vi "CRYGraph Get.vi"(11 "pGraph VI In":refnum<vi>) -> (3 "Graph Cluster":T1)   [LabVIEW 2013]
uses:
  Control/CRYGraph Property.ctl
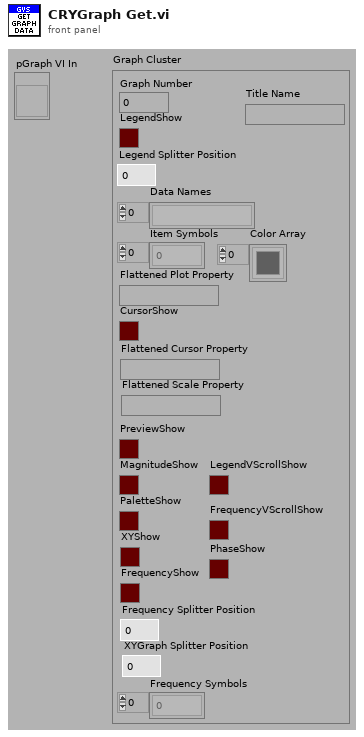
[diagram p1: front panel]
types:
  T1 = typedef "CRYGraph Property.ctl" = cluster{"LegendShow":bool, "Legend Splitter Position":dbl, "Data Names":string[], "Item Symbols":i32[], "Color Array":u32[], "Flattened Plot Property":string, "CursorShow":bool, "Flattened Cursor Property":string, "Graph Number":i32, "Flattened Scale Property":string, "PreviewShow":bool, "MagnitudeShow":bool, "PaletteShow":bool, "XYShow":bool, "FrequencyShow":bool, "Frequency Splitter Position":dbl, "XYGraph Splitter Position":dbl, "Frequency Symbols":i32[], "LegendVScrollShow":bool, "FrequencyVScrollShow":bool, "PhaseShow":bool, "Title Name":string}
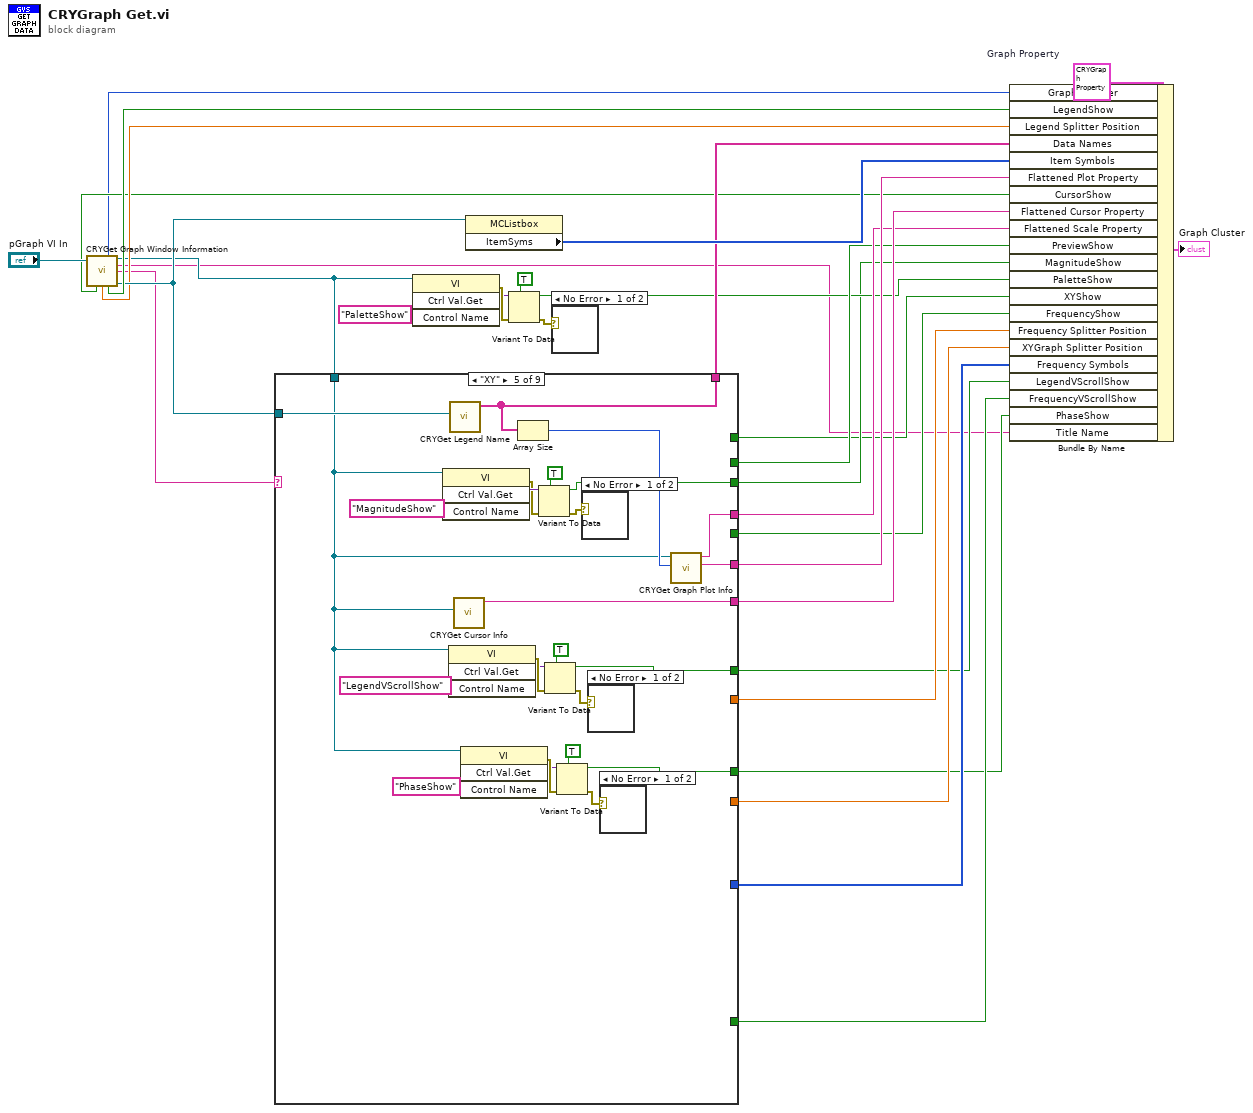
[diagram p0: block diagram]
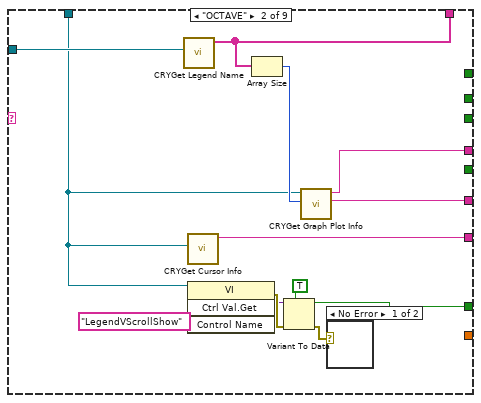
[diagram p4: hidden frame]
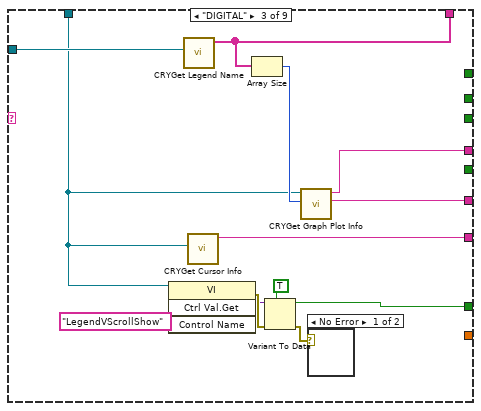
[diagram p6: hidden frame]
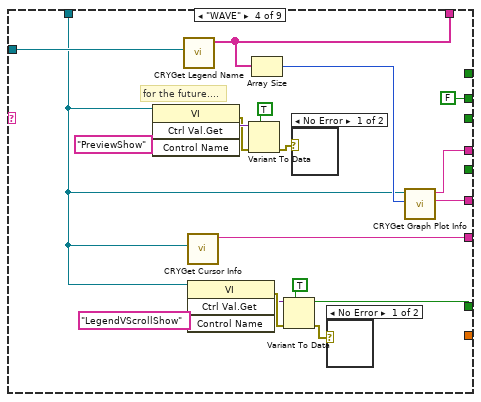
[diagram p8: hidden frame]
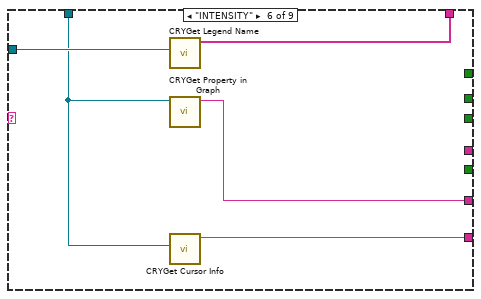
[diagram p14: hidden frame]
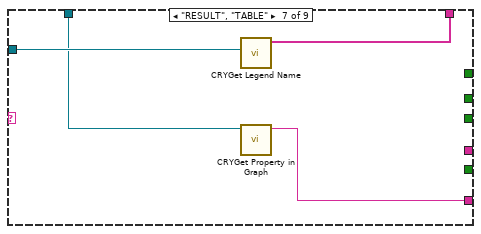
[diagram p15: hidden frame]
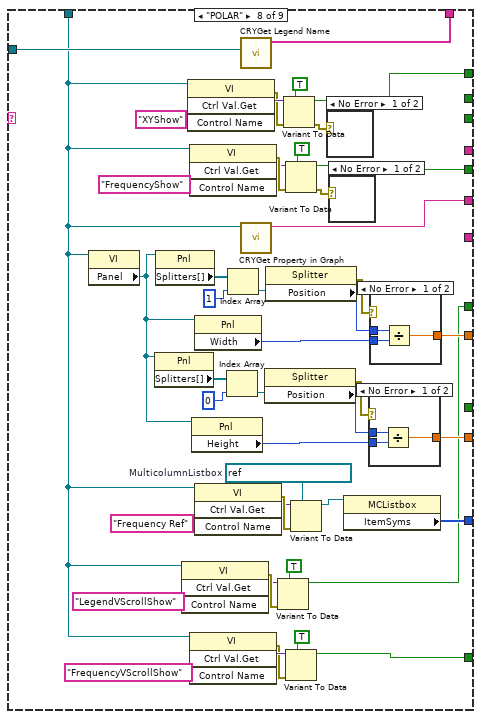
[diagram p16: hidden frame]
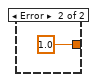
[diagram p17: hidden frame]
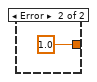
[diagram p18: hidden frame]
diagram:
  w32 = T1 {"LegendShow"=FALSE, "Legend Splitter Position"=0.0, "Data Names"=[], "Item Symbols"=[], "Color Array"=[], "Flattened Plot Property"="", "CursorShow"=FALSE, "Flattened Cursor Property"="", "Graph Number"=0, "Flattened Scale Property"="", "PreviewShow"=FALSE, "MagnitudeShow"=FALSE, "PaletteShow"=FALSE, "XYShow"=FALSE, "FrequencyShow"=FALSE, "Frequency Splitter Position"=0.0, "XYGraph Splitter Position"=0.0, "Frequency Symbols"=[], "LegendVScrollShow"=FALSE, "FrequencyVScrollShow"=FALSE, "PhaseShow"=FALSE, "Title Name"=""}  # Graph Property
  n1 = call "CRYGet Graph Window Information.vi"("pGraph VI In"="pGraph VI In") -> ("Graph Number Out"=w21:i32, "pGraph VI Out"=w9:refnum<vi>, "Garph Title Out"=w1:string, "Graph Type Out"=w10:string, "CursorShow Out"=w24:bool, "Legend Splitter Position"=w27:dbl, "LegendShow Out"=w30:bool, "Legend Ref Out"=w28:refnum<vi>)  [unwired: 2 in, 5 out]
  n2 = case shown="\"XY\"" w10 {
    tunnel: w28 -> [_ w45 w58 w77 w102 w107 w111 w158 _]
    tunnel: w9 -> [_ w33 w47 w60 w79 w103 w109 w113 w168]
    tunnel: [_ w44 w57 w76 w101 w106 w110 w157 _] -> w26
    tunnel: [_ w40 w53 w72 w97 w104 w108 w156 w167] -> w25
    tunnel: [_ w43 w56 w75 w100 w105 _ _ _] -> w23
    tunnel: [_ w42 w55 w74 w99 _ _ _ _] -> w22
    tunnel: [_ _ _ FALSE ("type") _ _ _ _ _] -> w20
    tunnel: [_ _ _ _ w91 _ _ _ _] -> w13
    tunnel: [_ _ _ _ _ _ _ w145 _] -> w11
    tunnel: [_ _ _ _ _ _ _ w144 _] -> w12
    tunnel: [_ _ _ _ _ _ _ w138 _] -> w8
    tunnel: [_ _ _ _ _ _ _ w131 _] -> w7
    tunnel: [_ _ _ _ _ _ _ w123 _] -> w6
    tunnel: [_ w34 w46 w59 w85 _ _ w118 _] -> w4
    tunnel: [_ _ _ _ _ _ _ w112 _] -> w3
    tunnel: [_ _ _ _ w78 _ _ _ _] -> w2
    frame Default {
    }
    frame "OCTAVE" {
      n3 = call "CRYGet Legend Name.vi"("MCListbox Refnum"=w45) -> ("Names Out"=w44:string[])  [unwired: 2 in, 8 out]
      n4 = call "CRYGet Cursor Info.vi"("pGraph VI"=w33) -> ("Flattened Cursor Property"=w43:string)  [unwired: 10 in]
      n5 = invoke class="VI" method="Ctrl Val.Get"(reference=w33, "Control Name"="LegendVScrollShow") -> (error out=w38:errorcluster, "Get Control Value Variant"=w36:variant)  [unwired: 2 in, 2 out]
      n6 = Array Size(array=w44) -> (size(s)=w41:i32)
      n7 = Variant To Data(error in=w38, type=TRUE, Variant=w36) -> (data=w34:bool, error out=w39:errorcluster)
      n8 = call "CRYGet Graph Plot Info.vi"("Plot Count"=w41, "Graph VI Ref"=w33) -> ("Flattened Plot Property"=w40:string, "Flattened Scale Property"=w42:string)  [unwired: 8 in]
      n9 = case shown="No Error" w39 {
        frame No Error {
        }
        frame Error {
        }
      }
    }
    frame "DIGITAL" {
      n10 = invoke class="VI" method="Ctrl Val.Get"(reference=w47, "Control Name"="LegendVScrollShow") -> (error out=w51:errorcluster, "Get Control Value Variant"=w49:variant)  [unwired: 2 in, 2 out]
      n11 = call "CRYGet Legend Name.vi"("MCListbox Refnum"=w58) -> ("Names Out"=w57:string[])  [unwired: 2 in, 8 out]
      n12 = call "CRYGet Cursor Info.vi"("pGraph VI"=w47) -> ("Flattened Cursor Property"=w56:string)  [unwired: 10 in]
      n13 = Array Size(array=w57) -> (size(s)=w54:i32)
      n14 = Variant To Data(error in=w51, type=TRUE, Variant=w49) -> (data=w46:bool, error out=w52:errorcluster)
      n15 = call "CRYGet Graph Plot Info.vi"("Plot Count"=w54, "Graph VI Ref"=w47) -> ("Flattened Plot Property"=w53:string, "Flattened Scale Property"=w55:string)  [unwired: 8 in]
      n16 = case shown="No Error" w52 {
        frame No Error {
        }
        frame Error {
        }
      }
    }
    frame "WAVE" {
      # "for the future...."
      n17 = invoke class="VI" method="Ctrl Val.Get"(reference=w60, "Control Name"="PreviewShow") -> (error out=w68:errorcluster, "Get Control Value Variant"=w70:variant)  [unwired: 2 in, 2 out]
      n18 = call "CRYGet Legend Name.vi"("MCListbox Refnum"=w77) -> ("Names Out"=w76:string[])  [unwired: 2 in, 8 out]
      n19 = call "CRYGet Cursor Info.vi"("pGraph VI"=w60) -> ("Flattened Cursor Property"=w75:string)  [unwired: 10 in]
      n20 = invoke class="VI" method="Ctrl Val.Get"(reference=w60, "Control Name"="LegendVScrollShow") -> (error out=w64:errorcluster, "Get Control Value Variant"=w62:variant)  [unwired: 2 in, 2 out]
      n21 = Variant To Data(error in=w68, type=TRUE, Variant=w70) -> (error out=w67:errorcluster)  [unwired: 1 out]
      n22 = Array Size(array=w76) -> (size(s)=w73:i32)
      n23 = Variant To Data(error in=w64, type=TRUE, Variant=w62) -> (data=w59:bool, error out=w65:errorcluster)
      n24 = case shown="No Error" w67 {
        frame No Error {
        }
        frame Error {
        }
      }
      n25 = case shown="No Error" w65 {
        frame No Error {
        }
        frame Error {
        }
      }
      n26 = call "CRYGet Graph Plot Info.vi"("Plot Count"=w73, "Graph VI Ref"=w60) -> ("Flattened Plot Property"=w72:string, "Flattened Scale Property"=w74:string)  [unwired: 8 in]
    }
    frame "XY" {
      n27 = invoke class="VI" method="Ctrl Val.Get"(reference=w79, "Control Name"="MagnitudeShow") -> (error out=w93:errorcluster, "Get Control Value Variant"=w95:variant)  [unwired: 2 in, 2 out]
      n28 = invoke class="VI" method="Ctrl Val.Get"(reference=w79, "Control Name"="LegendVScrollShow") -> (error out=w89:errorcluster, "Get Control Value Variant"=w87:variant)  [unwired: 2 in, 2 out]
      n29 = call "CRYGet Legend Name.vi"("MCListbox Refnum"=w102) -> ("Names Out"=w101:string[])  [unwired: 2 in, 8 out]
      n30 = call "CRYGet Cursor Info.vi"("pGraph VI"=w79) -> ("Flattened Cursor Property"=w100:string)  [unwired: 10 in]
      n31 = invoke class="VI" method="Ctrl Val.Get"(reference=w79, "Control Name"="PhaseShow") -> (error out=w83:errorcluster, "Get Control Value Variant"=w81:variant)  [unwired: 2 in, 2 out]
      n32 = Array Size(array=w101) -> (size(s)=w98:i32)
      n33 = Variant To Data(error in=w93, type=TRUE, Variant=w95) -> (data=w91:bool, error out=w92:errorcluster)
      n34 = Variant To Data(error in=w89, type=TRUE, Variant=w87) -> (data=w85:bool, error out=w90:errorcluster)
      n35 = Variant To Data(error in=w83, type=TRUE, Variant=w81) -> (data=w78:bool, error out=w84:errorcluster)
      n36 = case shown="No Error" w92 {
        frame No Error {
        }
        frame Error {
        }
      }
      n37 = case shown="No Error" w90 {
        frame No Error {
        }
        frame Error {
        }
      }
      n38 = case shown="No Error" w84 {
        frame No Error {
        }
        frame Error {
        }
      }
      n39 = call "CRYGet Graph Plot Info.vi"("Plot Count"=w98, "Graph VI Ref"=w79) -> ("Flattened Plot Property"=w97:string, "Flattened Scale Property"=w99:string)  [unwired: 8 in]
    }
    frame "INTENSITY" {
      n40 = call "CRYGet Legend Name.vi"("MCListbox Refnum"=w107) -> ("Names Out"=w106:string[])  [unwired: 2 in, 8 out]
      n41 = call "CRYGet Property in Graph.vi"("Graph VI Ref"=w103) -> ("Flattened Property"=w104:string)  [unwired: 10 in]
      n42 = call "CRYGet Cursor Info.vi"("pGraph VI"=w103) -> ("Flattened Cursor Property"=w105:string)  [unwired: 10 in]
    }
    frame "RESULT", "TABLE" {
      n43 = call "CRYGet Legend Name.vi"("MCListbox Refnum"=w111) -> ("Names Out"=w110:string[])  [unwired: 2 in, 8 out]
      n44 = call "CRYGet Property in Graph.vi"("Graph VI Ref"=w109) -> ("Flattened Property"=w108:string)  [unwired: 10 in]
    }
    frame "POLAR" {
      w142 = refnum<vi> refnum  # MulticolumnListbox
      n45 = property class="VI"(reference=w113) -> ("Panel"=w124:refnum<vi>)  [unwired: 1 in, 2 out]
      n46 = property class="Pnl"(reference=w124) -> ("Splitters[]"=w130:refnum<vi>[])  [unwired: 1 in, 2 out]
      n47 = property class="Pnl"(reference=w124) -> ("Splitters[]"=w132:refnum<vi>[])  [unwired: 1 in, 2 out]
      n48 = invoke class="VI" method="Ctrl Val.Get"(reference=w113, "Control Name"="LegendVScrollShow") -> (error out=w122:errorcluster, "Get Control Value Variant"=w120:variant)  [unwired: 2 in, 2 out]
      n49 = invoke class="VI" method="Ctrl Val.Get"(reference=w113, "Control Name"="XYShow") -> (error out=w152:errorcluster, "Get Control Value Variant"=w154:variant)  [unwired: 2 in, 2 out]
      n50 = invoke class="VI" method="Ctrl Val.Get"(reference=w113, "Control Name"="FrequencyShow") -> (error out=w149:errorcluster, "Get Control Value Variant"=w147:variant)  [unwired: 2 in, 2 out]
      n51 = invoke class="VI" method="Ctrl Val.Get"(reference=w113, "Control Name"="FrequencyVScrollShow") -> (error out=w114:errorcluster, "Get Control Value Variant"=w116:variant)  [unwired: 2 in, 2 out]
      n52 = property class="Pnl"(reference=w124) -> ("Height"=w127:u32)  [unwired: 1 in, 2 out]
      n53 = property class="Pnl"(reference=w124) -> ("Width"=w135:u32)  [unwired: 1 in, 2 out]
      n54 = invoke class="VI" method="Ctrl Val.Get"(reference=w113, "Control Name"="Frequency Ref") -> (error out=w141:errorcluster, "Get Control Value Variant"=w140:variant)  [unwired: 2 in, 2 out]
      n55 = Index Array(array=w130, index=0) -> (element=w128:refnum<vi>)
      n56 = Index Array(array=w132, index=1) -> (element=w134:refnum<vi>)
      n57 = call "CRYGet Legend Name.vi"("MCListbox Refnum"=w158) -> ("Names Out"=w157:string[])  [unwired: 2 in, 8 out]
      n58 = call "CRYGet Property in Graph.vi"("Graph VI Ref"=w113) -> ("Flattened Property"=w156:string)  [unwired: 10 in]
      n59 = property class="Splitter"(reference=w128) -> (error out=w125:errorcluster, "Position"=w126:i32)  [unwired: 1 in, 1 out]
      n60 = property class="Splitter"(reference=w134) -> (error out=w137:errorcluster, "Position"=w136:i32)  [unwired: 1 in, 1 out]
      n61 = Variant To Data(error in=w122, type=TRUE, Variant=w120) -> (data=w118:bool)  [unwired: 1 out]
      n62 = Variant To Data(error in=w152, type=TRUE, Variant=w154) -> (data=w144:bool, error out=w151:errorcluster)
      n63 = Variant To Data(error in=w149, type=TRUE, Variant=w147) -> (data=w145:bool, error out=w150:errorcluster)
      n64 = Variant To Data(error in=w114, type=TRUE, Variant=w116) -> (data=w112:bool)  [unwired: 1 out]
      n65 = Variant To Data(error in=w141, type=w142, Variant=w140) -> (data=w143:refnum<vi>)  [unwired: 1 out]
      n66 = case shown="No Error" w151 {
        frame No Error {
        }
        frame Error {
        }
      }
      n67 = case shown="No Error" w150 {
        frame No Error {
        }
        frame Error {
        }
      }
      n68 = property class="MCListbox"(reference=w143) -> ("ItemSyms"=w138:i32[])  [unwired: 1 in, 2 out]
      n69 = case shown="No Error" w125 {
        tunnel: [w161 1.0] -> w123
        tunnel: w127 -> [w160 _]
        tunnel: w126 -> [w159 _]
        frame No Error {
          n70 = Divide(x=w159, y=w160) -> (x/y=w161:dbl)
        }
        frame Error {
        }
      }
      n71 = case shown="No Error" w137 {
        tunnel: [w165 1.0] -> w131
        tunnel: w135 -> [w164 _]
        tunnel: w136 -> [w163 _]
        frame No Error {
          n72 = Divide(x=w163, y=w164) -> (x/y=w165:dbl)
        }
        frame Error {
        }
      }
    }
    frame "PICTURE", "TEXT" {
      n73 = call "CRYGet Property in Graph.vi"("Graph VI Ref"=w168) -> ("Flattened Property"=w167:string)  [unwired: 10 in]
    }
  }
  n74 = invoke class="VI" method="Ctrl Val.Get"(reference=w9, "Control Name"="PaletteShow") -> (error out=w18:errorcluster, "Get Control Value Variant"=w16:variant)  [unwired: 2 in, 2 out]
  n75 = property class="MCListbox"(reference=w28) -> ("ItemSyms"=w29:i32[])  [unwired: 1 in, 2 out]
  n76 = Variant To Data(error in=w18, type=TRUE, Variant=w16) -> (data=w14:bool, error out=w19:errorcluster)
  n77 = case shown="No Error" w19 {
    frame No Error {
    }
    frame Error {
    }
  }
  n78 = Bundle By Name(cluster=w32, "Graph Number"=w21, "LegendShow"=w30, "Legend Splitter Position"=w27, "Data Names"=w26, "Item Symbols"=w29, "Flattened Plot Property"=w25, "CursorShow"=w24, "Flattened Cursor Property"=w23, "Flattened Scale Property"=w22, "PreviewShow"=w20, "MagnitudeShow"=w13, "PaletteShow"=w14, "XYShow"=w12, "FrequencyShow"=w11, "Frequency Splitter Position"=w7, "XYGraph Splitter Position"=w6, "Frequency Symbols"=w8, "LegendVScrollShow"=w4, "FrequencyVScrollShow"=w3, "PhaseShow"=w2, "Title Name"=w1) -> (→"Graph Cluster":T1)
